vi "TSCAN_EnableReceive.vi"(8 "错误输入（无错误）":errorcluster, 11 "路径输入":path) -> (0 "错误输出":errorcluster, 3 "路径输出":path)   [LabVIEW 2019]
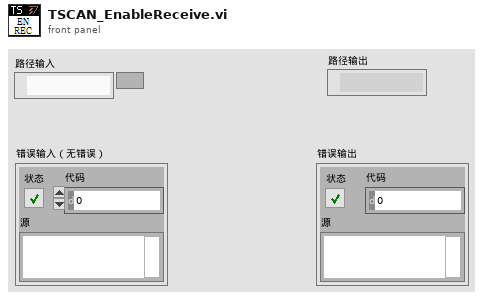
[diagram p1: front panel]
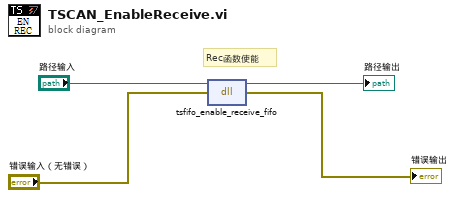
[diagram p0: block diagram]
diagram:
  # "Rec函数使能"
  n1 = dll-call lib="PTH2Habs CUsers\nAdministratorDesktopTS_Can通讯PathTSMaster.dll" fn="tsfifo_enable_receive_fifo"(path in="路径输入", error in="错误输入（无错误）") -> (path out=→"路径输出":path, error out=→"错误输出":errorcluster)  [unwired: 2 in]
